vi "Resistor Calculator 2012 NIVerified.vi"(9 "Color Band 3":T1=11 items=["Black"=0, "Brown"=1, "Red"=2, "Orange"=3, "Yellow"=4, "Green"=5, "Blue"=6, "Violet"=7, "Grey"=8, "White"=9, "Please Select"=11], 10 "Color Band 2":T1=11 items=["Black"=0, "Brown"=1, "Red"=2, "Orange"=3, "Yellow"=4, "Green"=5, "Blue"=6, "Violet"=7, "Grey"=8, "White"=9, "Please Select"=11], 11 "Color Band 1":T1=11 items=["Black"=0, "Brown"=1, "Red"=2, "Orange"=3, "Yellow"=4, "Green"=5, "Blue"=6, "Violet"=7, "Grey"=8, "White"=9, "Please Select"=11]) -> (2 "Invalid Color":bool, 3 "Resistor Value":dbl)   [LabVIEW 2012]
uses:
  Colors.ctl
panel:
  in  "Stop":bool
  # "Overview: This example calculates the theoretical value of the resistor based on the supplied band colors.\nRequirements: LabVIEW Base Development System\nInstructions:\n1- Run the VI\n2- Select the values of bands 1-3 from drop down menu\n3- the Resistor Value changes when changing the bands colors\n4- If the user doesn't select any color, the output will be (-1) and Invalid Color LED will turn ON"
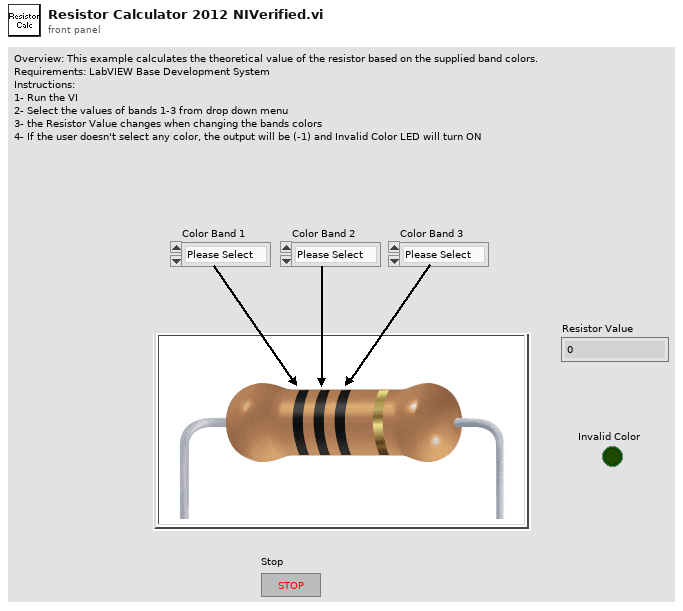
[diagram p1: front panel]
types:
  T1 = typedef "Colors.ctl" = u16
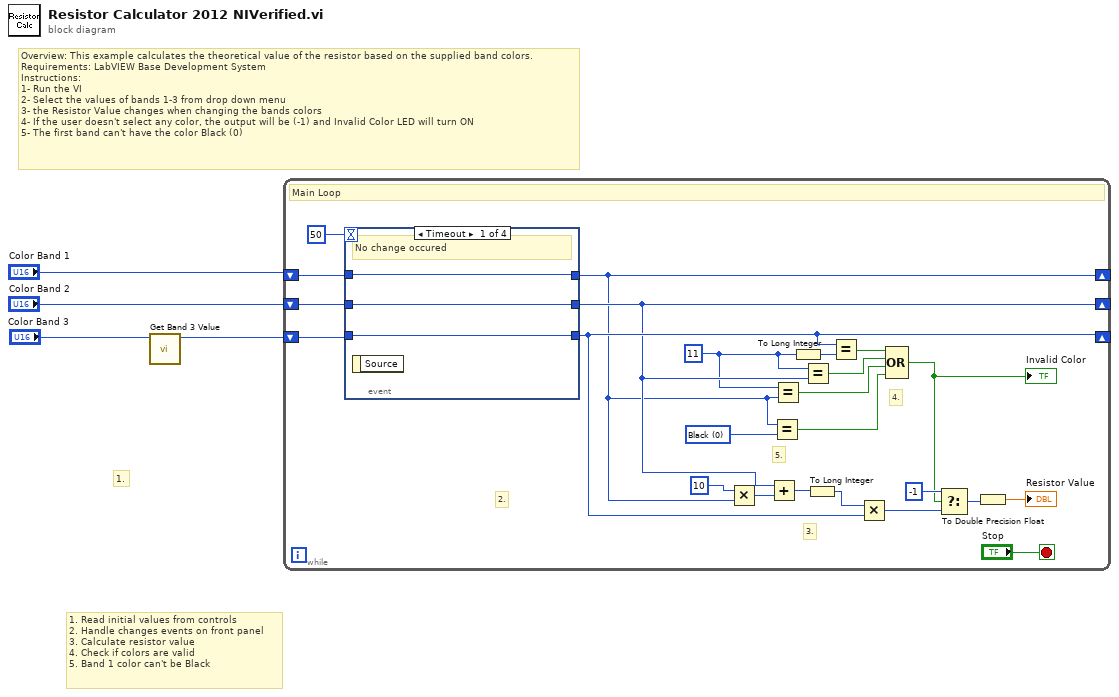
[diagram p0: block diagram]
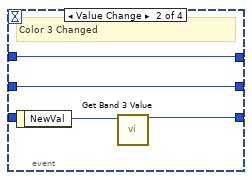
[diagram p2: hidden frame]
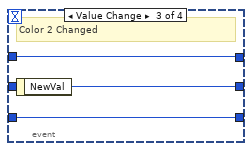
[diagram p3: hidden frame]
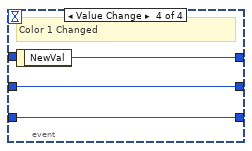
[diagram p4: hidden frame]
diagram:
  # "Overview: This example calculates the theoretical value of the resistor based on the supplied band colors.\nRequirements: LabVIEW Base Development System\nInstructions:\n1- Run the VI\n2- Select the values of bands 1-3 from drop down menu\n3- the Resistor Value changes when changing the bands colors\n4- If the user doesn't select any color, the output will be (-1) and Invalid Color LED will turn ON\n5- The first band can't have the color Black (0)"
  # "1. Read initial values from controls\n2. Handle changes events on front panel\n3. Calculate resistor value\n4. Check if colors are valid\n5. Band 1 color can't be Black"
  # "1."
  n1 = call "Get Band 3 Value.vi"("Color Band 3"="Color Band 3") -> ("Multiplier"=w3:i32)  [unwired: 10 in]
  n2 = while {
    shift-right: [w5] -> _
    shift-left: "Color Band 1" -> [w25]
    shift-right: [w11] -> _
    shift-left: "Color Band 2" -> [w24]
    shift-right: [w17] -> _
    shift-left: w3 -> [w23]
    stop <- "Stop" stop-if-true
    w7 = T1 0 items=["Black"=0, "Brown"=1, "Red"=2, "Orange"=3, "Yellow"=4, "Green"=5, "Blue"=6, "Violet"=7, "Grey"=8, "White"=9, "Please Select"=11] ("y")
    w9 = u16 11 ("y")
    # "5."
    # "4."
    # "3."
    # "2."
    # "Main Loop"
    n3 = event shown="[0] Timeout" {
      selector: _ -> [_ _ _ _]
      dyn-events: _ -> [_ _ _ _]
      timeout: 50 -> [_ _ _ _]
      tunnel: [w31 w34 w37 w39] -> w5
      tunnel: [w30 w35 w36 w40] -> w11
      tunnel: [w29 w32 w38 w41] -> w17
      tunnel: w25 -> [w31 w34 w37 _]
      tunnel: w24 -> [w30 w35 _ w40]
      tunnel: w23 -> [w29 _ w38 w41]
      event Timeout {
        # "No change occured"
        n4 = event-data() -> ()  [unwired: 1 in, 1 out]
      }
      event Value Change {
        # "Color 3 Changed"
        n5 = event-data() -> ("NewVal"=w33:T1)  [unwired: 1 in]
        n6 = call "Get Band 3 Value.vi"("Color Band 3"=w33) -> ("Multiplier"=w32:i32)  [unwired: 10 in]
      }
      event Value Change {
        # "Color 2 Changed"
        n7 = event-data() -> ("NewVal"=w36:T1)  [unwired: 1 in]
      }
      event Value Change {
        # "Color 1 Changed"
        n8 = event-data() -> ("NewVal"=w39:T1)  [unwired: 1 in]
      }
    }
    n9 = Multiply(x=u16 10 ("y"), y=w5) -> (x*y=w28:T1)
    n10 = Add(x=w11, y=w28) -> (x+y=w14:T1)
    n11 = Equal?(x=w5, y=w7) -> (x = y?=w6:bool)
    n12 = Equal?(x=w9, y=w5) -> (x = y?=w8:bool)
    n13 = To Long Integer(number=w9) -> (32bit integer=w12:i32)
    n14 = Equal?(x=w9, y=w11) -> (x = y?=w16:bool)
    n15 = To Long Integer(number=w14) -> (32bit integer=w13:i32)
    n16 = Equal?(x=w17, y=w12) -> (x = y?=w15:bool)
    n17 = Multiply(x=w13, y=w17) -> (x*y=w21:i32)
    n18 = Compound Arithmetic op=OR(w15, w16, w8, w6) -> (w18:bool)
    "Invalid Color" <- w18
    n19 = Select(t=-1, s=w18, f=w21) -> (s? t:f=w20:i32)
    n20 = To Double Precision Float(number=w20) -> (double precision float=→"Resistor Value":dbl)
  }
